vi "LoadTabControl.vi"(10 "Control in":refnum<vi>, 11 "Array in":T1[](array[typedef])) -> (3 "Array out":T1[](array[typedef]))   [LabVIEW 2017, in "ContextHelpEditor.lvlib"]
uses:
  ContextHelpEditor.lvlib
  TabbedControl--cluster.ctl
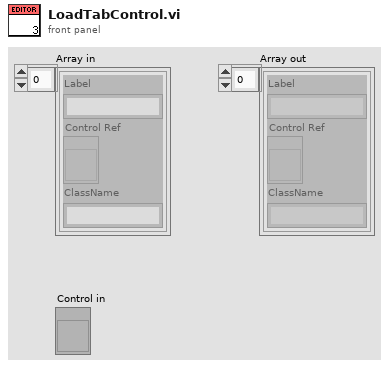
[diagram p1: front panel]
types:
  T1 = typedef "ContextHelpEditor.lvlib/TabbedControl--cluster.ctl" = cluster{"Label":string, "Control Ref":refnum<vi>, "ClassName":string}
  T2 = enum8{"Enabled", "Disabled", "Disabled and Grayed Out"}
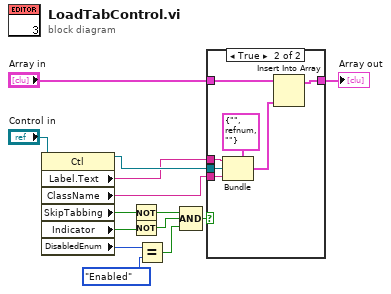
[diagram p0: block diagram]
diagram:
  n1 = property class="Ctl"(reference="Control in") -> (reference out=w14:refnum<vi>, "Label.Text"=w12:string, "ClassName"=w13:string, "SkipTabbing"=w2:bool, "Indicator"=w3:bool, "DisabledEnum"=w4:T2)  [unwired: 1 in, 1 out]
  n2 = Not(x=w2) -> (.not. x?=w6:bool)
  n3 = Not(x=w3) -> (.not. x?=w7:bool)
  n4 = Equal?(x=w4, y=T2."Enabled") -> (x = y?=w8:bool)
  n5 = Compound Arithmetic op=AND(w6, w7, w8) -> (w9:bool)
  n6 = case shown="True" w9 {
    tunnel: w12 -> [_ w21]
    tunnel: w14 -> [_ w20]
    tunnel: w13 -> [_ w19]
    tunnel: "Array in" -> [w15 w18]
    tunnel: [w15 w17] -> w11
    frame False {
    }
    frame True {
      n7 = Bundle(cluster=T1 {"Label"="", "Control Ref"=refnum, "ClassName"=""} ("TabbedControl"), "Label"=w21, "Control Ref"=w20, "ClassName"=w19) -> (w16:T1)
      n8 = Insert Into Array(array=w18, new element=w16) -> (w17:T1[])  [unwired: 1 in]
    }
  }
  "Array out" <- w11
